vi "Tx Message to Map Value.vi"(8 "error in":errorcluster, 10 "message":T2={"name"="", "message type"="BC to RT", "endpoint Rx"={"terminal address"=0, "subaddress"=0}, "endpoint Tx"={"terminal address"=0, "subaddress"=0}, "mode code"=0, "number of words"=0, "parameters"=[], "create timestamp channel"=FALSE}, 11 "remote terminal handles":u64[](array[numeric])) -> (0 "error out":errorcluster, 3 "Tx write info":T1)   [LabVIEW 2020, in "Ballard MIL-STD-1553 Engine.lvlib" / "Custom Device.lvlib"]
uses:
  Custom Device.lvlib
  Shared/Message Definition.ctl
  Shared/Message Type.ctl
  Shared/Terminal Endpoint.ctl
  Shared/Address.ctl
  Shared/Parameter Definition.ctl
  Shared/Tx Write Info.ctl
  <instrlib>/BTI1553Lib/Public/Controls/1553 Transfer Direction.ctl
  <instrlib>/BTI1553Lib/Public/Controls/1553 RT Transfer Type.ctl
  <instrlib>/BTI1553Lib/Private/RT/Configure/Get RT Xfer Handle.vi
  <instrlib>/BTI1553Lib/BTI1553LV.lvlib
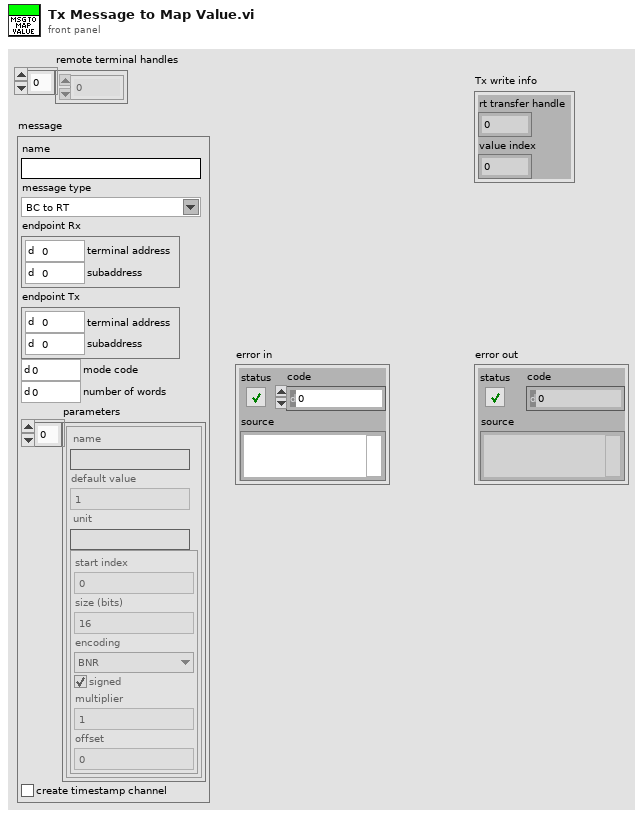
[diagram p1: front panel]
types:
  T1 = typedef "Tx Write Info.ctl" = cluster{"rt transfer handle":u64, "value index":i32}
  T2 = typedef "Message Definition.ctl" = cluster{"name":string, "message type":T3, "endpoint Rx":T4, "endpoint Tx":T4, "mode code":u16, "number of words":u16, "parameters":cluster{"name":string, "default value":dbl, "unit":string, "parameter definition":T6}[], "create timestamp channel":bool}
  T3 = typedef "Message Type.ctl" = string
  T4 = typedef "Terminal Endpoint.ctl" = cluster{"terminal address":T5, "subaddress":T5}
  T5 = typedef "Address.ctl" = u16
  T6 = typedef "Parameter Definition.ctl" = cluster{"start index":i32, "size (bits)":i32, "encoding":enum16{"BNR", "BCD", "Discrete"}, "signed":bool, "multiplier":dbl, "offset":dbl}
  T7 = typedef "BTI1553LV.lvlib/1553 Transfer Direction.ctl" = u32
  T8 = typedef "BTI1553LV.lvlib/1553 RT Transfer Type.ctl" = u32
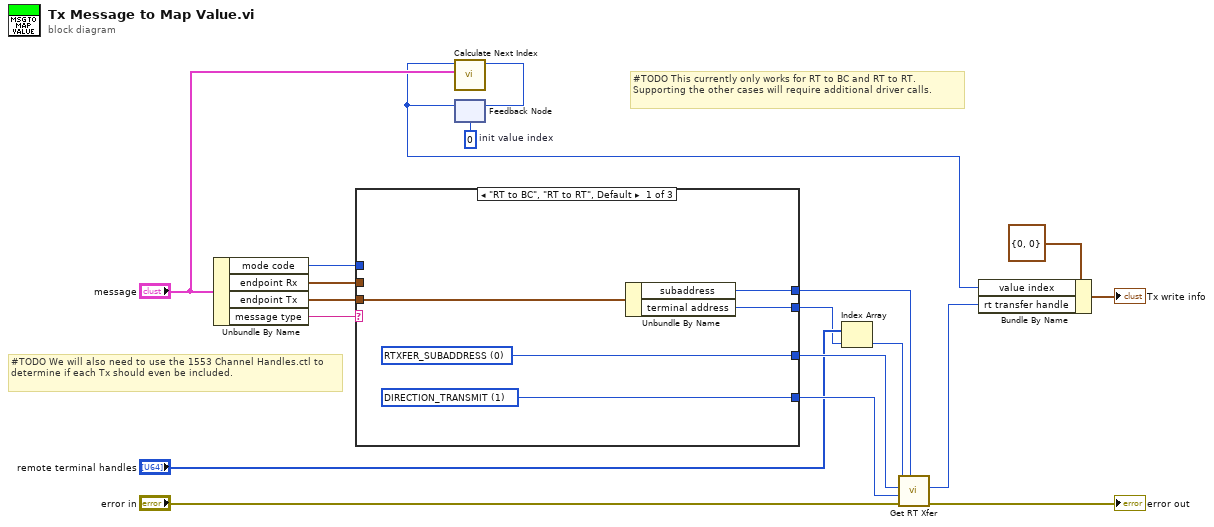
[diagram p0: block diagram]
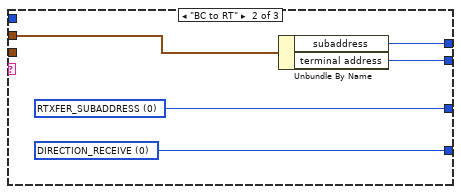
[diagram p2: hidden frame]
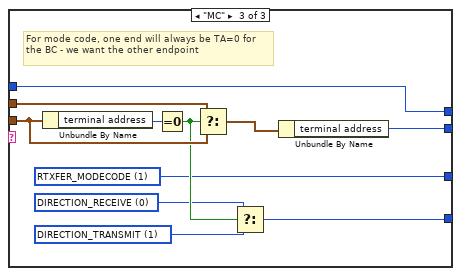
[diagram p3: hidden frame]
diagram:
  w5 = 0  # init value index
  # "#TODO We will also need to use the 1553 Channel Handles.ctl to determine if each Tx should even be included."
  # "#TODO This currently only works for RT to BC and RT to RT. Supporting the other cases will require additional driver calls."
  n1 = Unbundle By Name("message") -> ("mode code"=w1:u16, "endpoint Rx"=w19:T4, "endpoint Tx"=w18:T4, "message type"=w8:T3)
  n2 = case shown="\"RT to BC\", \"RT to RT\", Default" w8 {
    tunnel: w19 -> [_ w27 w39]
    tunnel: w18 -> [w22 _ w38]
    tunnel: [w24 w29 w34] -> w14
    tunnel: [w23 w28 w33] -> w13
    tunnel: [w21 w26 w30] -> w3
    tunnel: [w20 w25 w31] -> w2
    tunnel: w1 -> [_ _ w30]
    frame "RT to BC", "RT to RT", Default {
      w24 = T7 1 items=["DIRECTION_RECEIVE", "DIRECTION_TRANSMIT"] ("transfer direction")
      w23 = T8 0 items=["RTXFER_SUBADDRESS", "RTXFER_MODECODE"] ("transfer type")
      n3 = Unbundle By Name(w22) -> ("subaddress"=w21:T5, "terminal address"=w20:T5)
    }
    frame "BC to RT" {
      w29 = T7 0 items=["DIRECTION_RECEIVE", "DIRECTION_TRANSMIT"] ("transfer direction")
      w28 = T8 0 items=["RTXFER_SUBADDRESS", "RTXFER_MODECODE"] ("transfer type")
      n4 = Unbundle By Name(w27) -> ("subaddress"=w26:T5, "terminal address"=w25:T5)
    }
    frame "MC" {
      w35 = T7 1 items=["DIRECTION_RECEIVE", "DIRECTION_TRANSMIT"] ("transfer direction")
      w36 = T7 0 items=["DIRECTION_RECEIVE", "DIRECTION_TRANSMIT"] ("transfer direction")
      w33 = T8 1 items=["RTXFER_SUBADDRESS", "RTXFER_MODECODE"] ("transfer type")
      # "For mode code, one end will always be TA=0 for the BC - we want the other endpoint"
      n5 = Unbundle By Name(w38) -> ("terminal address"=w40:T5)
      n6 = Equal To 0?(x=w40) -> (x = 0?=w37:bool)
      n7 = Select(t=w39, s=w37, f=w38) -> (s? t:f=w32:T4)
      n8 = Select(t=w36, s=w37, f=w35) -> (s? t:f=w34:T7)
      n9 = Unbundle By Name(w32) -> ("terminal address"=w31:T5)
    }
  }
  n10 = feedback #1(w5) -> (w4:i32)
  n11 = call "Calculate Next Index.vi"("message"="message", "index"=w4) -> ("next index"=w6:i32)  [unwired: 9 in]
  n12 = feedback-in #1(w6) -> ()
  n13 = Index Array(array="remote terminal handles", index=w2) -> (element=w10:u64)
  n14 = call-poly <instrlib>:"Get RT Xfer.vi"("transfer sa number or mc number"=w3, "error in (no error)"="error in", "transfer direction"=w14, "transfer type"=w13, "remote terminal handle in"=w10) -> ("error out"=→"error out":errorcluster, "rt transfer handle out"=w12:u64)  [unwired: 4 in, 1 out]
  n15 = Bundle By Name(cluster=T1 {"rt transfer handle"=0, "value index"=0} ("Tx write info"), "value index"=w4, "rt transfer handle"=w12) -> (→"Tx write info":T1)
